vi "GetEvtReports.vi"(8 "error in (no error)":errorcluster, 11 "RingdownEvtPlugin in":refnum<class "RingdownEvtPlugin.lvclass">) -> (0 "error out":errorcluster, 3 "RingdownEvtPlugin out":refnum<class "RingdownEvtPlugin.lvclass">)   [LabVIEW 2014, in "EventPlugins.lvlib" / "RingdownEvtPlugin.lvclass"]
uses:
  RingdownEvtPlugin.lvclass
  EventPluginBaseClass/EventPluginBaseClass.lvclass/EventPluginBaseClass.ctl
  EventPluginBaseClass/TypeDefs/clEvtReport.ctl
  EventPluginBaseClass/Accessors/Read BusNumber.vi
  EventPluginBaseClass/Accessors/Read EvtConfig.vi
  EventPluginBaseClass/Accessors/Read TimeArray.vi
  EventPluginBaseClass/Accessors/Read EvtParams.vi
  EventPluginBaseClass/EventPluginBaseClass.lvclass
  C37EvtPlugin/C37EvtPlugin.lvclass
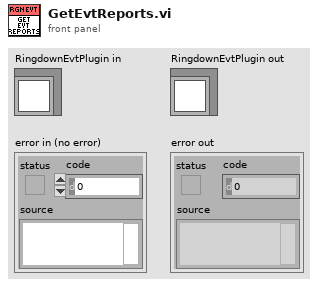
[diagram p1: front panel]
types:
  T1 = typedef "EventPlugins.lvlib/EventPluginBaseClass.lvclass/clEvtReport.ctl" = cluster{"Timestamp":dbl, "Synx":cdb[], "Freq":dbl, "ROCOF":dbl, "ID":i16}
  T2 = typedef "EventPlugins.lvlib/EventPluginBaseClass.lvclass/clEvtConfig.ctl" = cluster{"T0(UTC)":dbl, "F0":dbl, "Fs":i32, "FSamp":u32, "bPosSeq":bool}
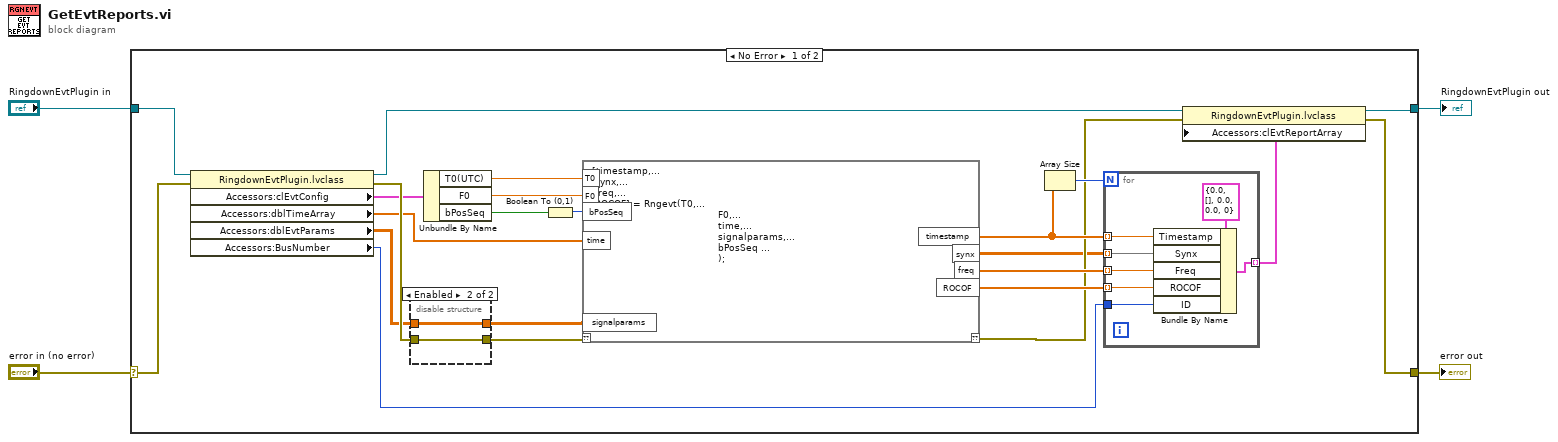
[diagram p0: block diagram]
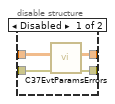
[diagram p2: hidden frame]
diagram:
  n1 = case shown="No Error" "error in (no error)" {
    selector: "error in (no error)" -> [w11 w42]
    tunnel: [w8 w42] -> w3
    tunnel: [w9 w41] -> w1
    tunnel: "RingdownEvtPlugin in" -> [w10 w41]
    frame No Error {
      n2 = property class="RingdownEvtPlugin.lvclass"(reference=w10, error in=w11) -> (reference out=w16:refnum<class "RingdownEvtPlugin.lvclass">, error out=w15:errorcluster, "Accessors:clEvtConfig"=w14:T2, "Accessors:dblTimeArray"=w13:dbl[], "Accessors:dblEvtParams"=w12:dbl[][], "Accessors:BusNumber"=w6:u8)
      n3 = disable-structure shown="Enabled" {
        disable-tunnel: [w31 w32] -> w18
        disable-tunnel: [w30 w33] -> w17
        disable-tunnel: w12 -> [w29 w33]
        disable-tunnel: w15 -> [w28 w32]
        frame Disabled {
          n4 = call "C37EvtParamsErrors.vi"("error in (no error)"=w28, "dblSignalParams in"=w29) -> ("error out"=w31:errorcluster, "dblSignalParams out"=w30:dbl[][])  [unwired: 8 in]
        }
        frame Enabled {
        }
      }
      n5 = Unbundle By Name(w14) -> ("T0(UTC)"=w25:dbl, "F0"=w24:dbl, "bPosSeq"=w7:bool)
      n6 = Boolean To (0,1)(Boolean=w7) -> (0, 1=w5:i16)
      n7 = script code="[timestamp,...\n synx,...\n freq,...\n ROCOF] = Rngevt(T0,...\n                                          F0,...\n                                          time,...\n                                          signalparams,...\n                                          bPosSeq ...\n                                          );"("??"=w18, "T0"=w25, "F0"=w24, "bPosSeq"=w5, "time"=w13, "signalparams"=w17) -> ("??"=w21:errorcluster, "timestamp"=w23:dbl[], "synx"=w20:cdb[][], "freq"=w27:dbl[], "ROCOF"=w26:dbl[])
      n8 = Array Size(array=w23) -> (size(s)=w22:i32)
      n9 = for {
        N: w22 -> [_]
        tunnel: w23 -> [w40] mode=indexing
        tunnel: w27 -> [w39] mode=indexing
        tunnel: w26 -> [w38] mode=indexing
        tunnel: [w36] -> w19 mode=indexing
        tunnel: w20 -> [w35] mode=indexing
        tunnel: w6 -> [w34]
        n10 = Bundle By Name(cluster=T1 {"Timestamp"=0.0, "Synx"=[], "Freq"=0.0, "ROCOF"=0.0, "ID"=0} ("clReport"), "Timestamp"=w40, "Synx"=w35, "Freq"=w39, "ROCOF"=w38, "ID"=w34) -> (w36:T1)
      }
      n11 = property class="RingdownEvtPlugin.lvclass"(reference=w16, error in=w21, "Accessors:clEvtReportArray"=w19) -> (reference out=w9:refnum<class "RingdownEvtPlugin.lvclass">, error out=w8:errorcluster)
    }
    frame Error {
    }
  }
  "error out" <- w3
  "RingdownEvtPlugin out" <- w1
